vi "sub UI set i.vi"(8 "error in (no error)":errorcluster, 10 "<i> data":T1, 11 "IDE simple in":refnum<class "LF2R IDE.lvclass">) -> (0 "error out":errorcluster, 3 "IDE simple out":refnum<class "LF2R IDE.lvclass">)   [LabVIEW 2018, in "LF2R IDE.lvlib" / "LF2R IDE.lvclass"]
uses:
  LF2R IDE.lvclass
  Frame Analizer/frame i data.ctl
  LF2R IDE.lvclass/LF2R IDE.ctl
  Frame Analizer/Data Parser.lvclass
panel:
  out "deleted portion":string[](array[string])
  out "Array":string[](array[string])
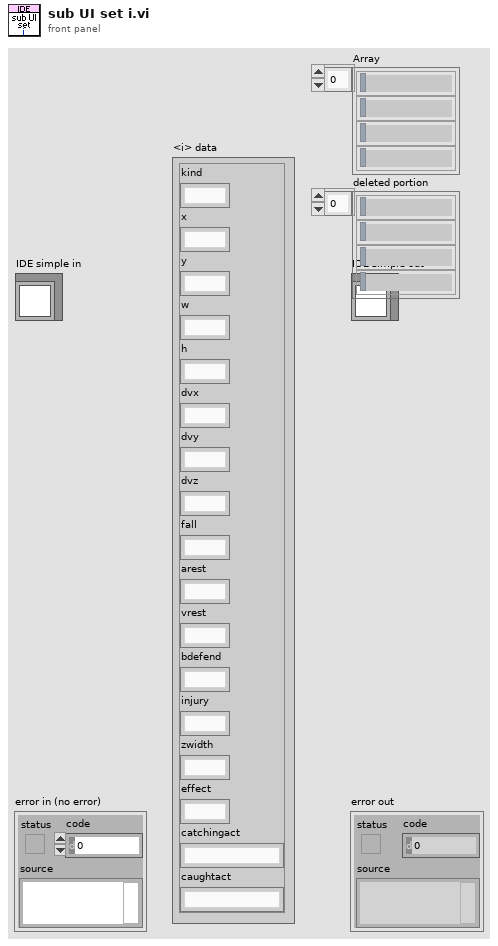
[diagram p1: front panel]
types:
  T1 = typedef "Data Parser.lvclass/frame i data.ctl" = cluster{"kind":string, "x":string, "y":string, "w":string, "h":string, "dvx":string, "dvy":string, "dvz":string, "fall":string, "arest":string, "vrest":string, "bdefend":string, "injury":string, "zwidth":string, "effect":string, "catchingact":string, "caughtact":string}
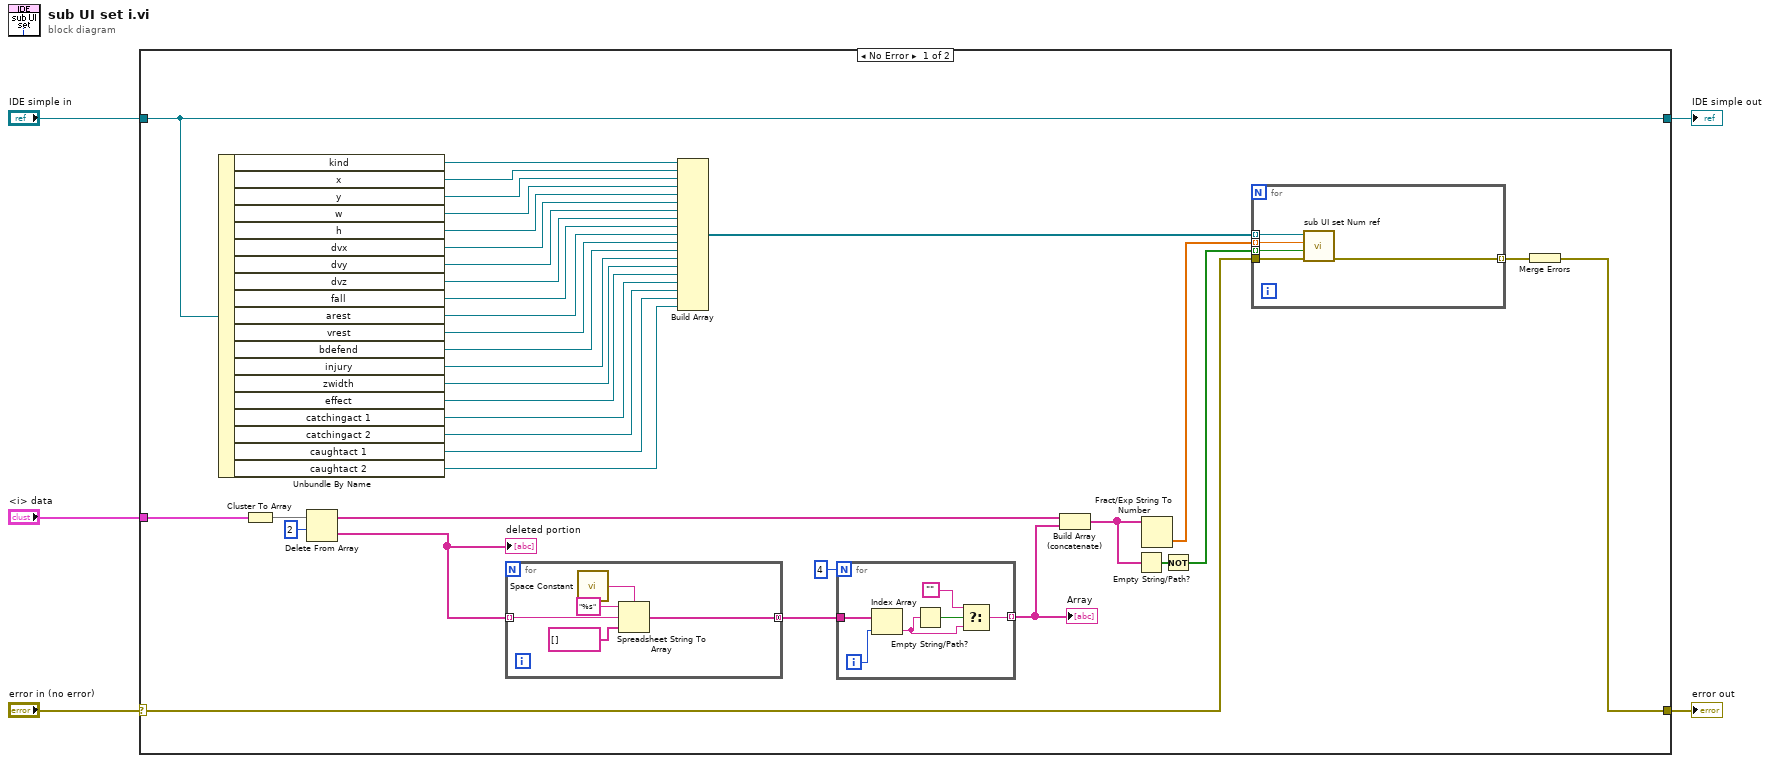
[diagram p0: block diagram]
diagram:
  n1 = case shown="No Error" "error in (no error)" {
    selector: "error in (no error)" -> [w40 w59]
    tunnel: [w35 w59] -> w4
    tunnel: [w37 w58] -> w2
    tunnel: "IDE simple in" -> [w37 w58]
    tunnel: "<i> data" -> [w34 _]
    frame No Error {
      n2 = Unbundle By Name(w37) -> ("kind"=w32:refnum<vi>, "x"=w31:refnum<vi>, "y"=w30:refnum<vi>, "w"=w29:refnum<vi>, "h"=w28:refnum<vi>, "dvx"=w27:refnum<vi>, "dvy"=w26:refnum<vi>, "dvz"=w25:refnum<vi>, "fall"=w24:refnum<vi>, "arest"=w23:refnum<vi>, "vrest"=w22:refnum<vi>, "bdefend"=w21:refnum<vi>, "injury"=w20:refnum<vi>, "zwidth"=w9:refnum<vi>, "effect"=w19:refnum<vi>, "catchingact 1"=w16:refnum<vi>, "catchingact 2"=w15:refnum<vi>, "caughtact 1"=w14:refnum<vi>, "caughtact 2"=w13:refnum<vi>)
      n3 = Cluster To Array(cluster=w34) -> (array=w17:string[])
      n4 = Delete From Array(array=w17, length=2) -> (deleted portion=w12:string[], array with subset deleted=w11:string[])  [unwired: 1 in]
      "deleted portion" <- w12
      n5 = for {
        tunnel: w12 -> [w52] mode=indexing
        tunnel: [w48] -> w8 mode=concatenating
        n6 = call <vilib>:"Space Constant.vi"() -> ("String"=w49:string)
        n7 = Spreadsheet String To Array(delimiter (Tab)=w49, format string="%s", spreadsheet string=w52, array type (2D Dbl)=string[] []) -> (array=w48:string[])
      }
      n8 = Build Array(w32, w31, w30, w29, w28, w27, w26, w25, w24, w23, w22, w21, w20, w9, w19, w16, w15, w14, w13) -> (w33:refnum<vi>[])
      n9 = for {
        N: 4 -> [_]
        tunnel: w8 -> [w45]
        tunnel: [w46] -> w6 mode=indexing
        i -> [w42]
        n10 = Index Array(array=w45, index=w42) -> (element=w43:string)
        n11 = Empty String/Path?(string/path=w43) -> (empty?=w44:bool)
        n12 = Select(t="", s=w44, f=w43) -> (s? t:f=w46:string)
      }
      "Array" <- w6
      n13 = Build Array (concatenate)(w11, w6) -> (w10:string[])
      n14 = Empty String/Path?(string/path=w10) -> (empty?=w41:bool[])
      n15 = Fract/Exp String To Number(string=w10) -> (number=w38:dbl[])  [unwired: 3 in, 1 out]
      n16 = Not(x=w41) -> (.not. x?=w39:bool[])
      n17 = for {
        tunnel: w40 -> [w57]
        tunnel: w33 -> [w53] mode=indexing
        tunnel: w39 -> [w54] mode=indexing
        tunnel: w38 -> [w56] mode=indexing
        tunnel: [w55] -> w36 mode=indexing
        n18 = call "sub UI set Num ref.vi"("error in"=w57, "valid"=w54, "Value"=w56, "num ref"=w53) -> ("error out"=w55:errorcluster)  [unwired: 7 in]
      }
      n19 = Merge Errors(w36) -> (w35:errorcluster)
    }
    frame Error {
    }
  }
  "error out" <- w4
  "IDE simple out" <- w2
